vi "BuildFarm Launcher.vi"() -> ()   [LabVIEW 2017]
uses:
  vi.lib/BenjaminR/Build Farm/Actors/BuildServer/BuildServer/BuildServer.lvclass
  C:/Users/Public/Documents/wc/BuildFarm/src/LabVIEW/vi.lib/BenjaminR/Build Farm/Actors/Framework/Actor wLauncher/Actor wLauncher.lvclass
  vi.lib/BenjaminR/Build Farm/Actors/Framework/Actor wLauncher/Actor wLauncher.lvclass
panel:
  out "Status":string caption="Launching BuildServer.lvlib:BuildServer.lvclass"
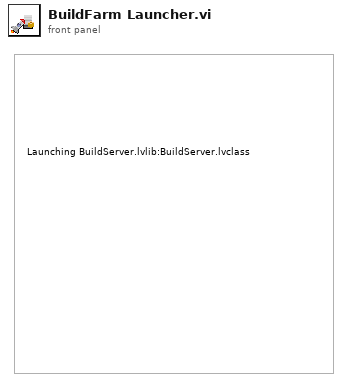
[diagram p1: front panel]
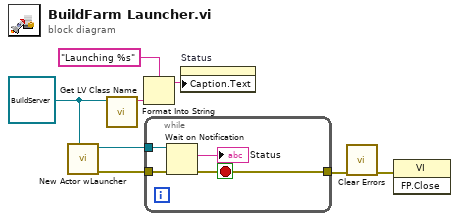
[diagram p0: block diagram]
diagram:
  w7 = refnum<class "BuildServer.lvclass"> refnum ("BuildServer.lvlib:BuildServer.lvclass")
  n1 = call "New Actor wLauncher.vi"("Actor wLauncher in"=w7) -> ("error out"=w1:errorcluster, "Launcher Notifier"=w8:refnum<notifier>)  [unwired: 8 in, 1 out]
  n2 = call <vilib>:"Get LV Class Name.vi"("object"=w7) -> ("class name"=w6:string)  [unwired: 9 in, 1 out]
  n3 = Format Into String(format string="Launching %s", w6) -> (resulting string=w5:string)  [unwired: 2 in, 1 out]
  n4 = while {
    tunnel: w8 -> [w12]
    tunnel: [w10] -> w3
    tunnel: w1 -> [w9]
    stop <- w10 stop-if-true
    n5 = Wait on Notification(notifier=w12, error in (no error)=w9) -> (notification=→"Status":string, error out=w10:errorcluster)  [unwired: 2 in, 2 out]
  }
  n6 = property on="Status" class="Str"("Caption.Text"=w5) -> ()  [unwired: 2 in, 2 out]
  n7 = call <vilib>:"Clear Errors.vi"("error in (no error)"=w3) -> ("error out"=w2:errorcluster)  [unwired: 5 in, 1 out]
  n8 = invoke class="VI" method="FP.Close"(error in=w2) -> ()  [unwired: 2 in, 3 out]
